vi "From Button Cluster To Button Table.vi"(8 "Error In":errorcluster, 11 "button info":T1) -> (0 "Error Out":errorcluster, 4 "Buttons array":bool[](array[boolean]), 5 "Which ones?":u8[](array[numeric]))   [LabVIEW 2014]
doc: "Converts buttons from joystick from cluster to table"
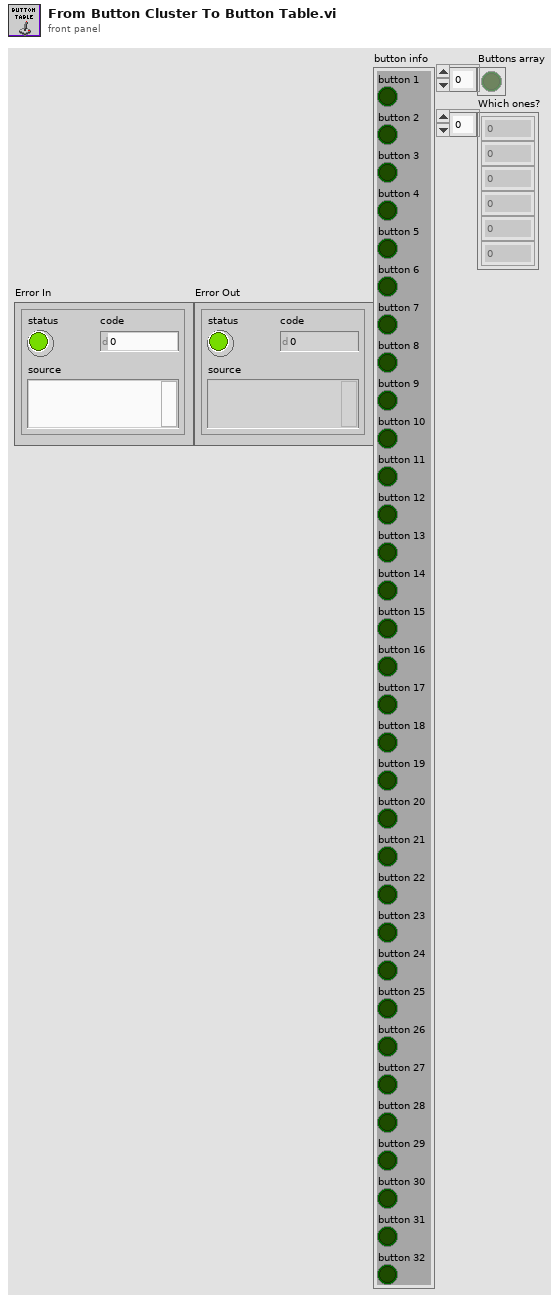
[diagram p1: front panel]
types:
  T1 = cluster{"button 1":bool, "button 2":bool, "button 3":bool, "button 4":bool, "button 5":bool, "button 6":bool, "button 7":bool, "button 8":bool, "button 9":bool, "button 10":bool, "button 11":bool, "button 12":bool, "button 13":bool, "button 14":bool, "button 15":bool, "button 16":bool, "button 17":bool, "button 18":bool, "button 19":bool, "button 20":bool, "button 21":bool, "button 22":bool, "button 23":bool, "button 24":bool, "button 25":bool, "button 26":bool, "button 27":bool, "button 28":bool, "button 29":bool, "button 30":bool, "button 31":bool, "button 32":bool}
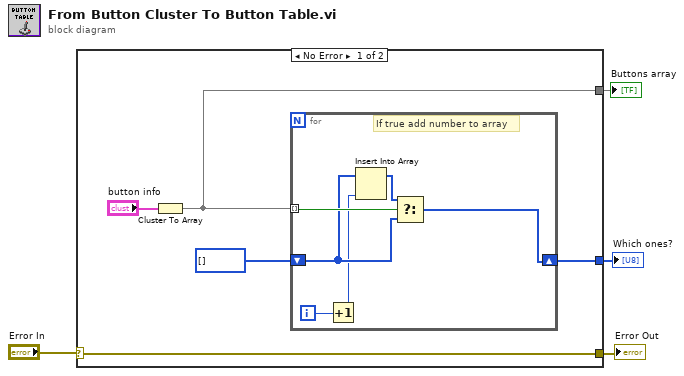
[diagram p0: block diagram]
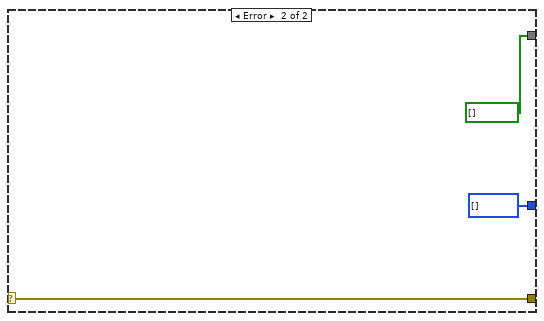
[diagram p2: hidden frame]
diagram:
  n1 = case shown="No Error" "Error In" {
    selector: "Error In" -> [w9 w18]
    tunnel: [w9 w18] -> w3
    tunnel: [w6 bool[] []] -> w2
    tunnel: [w5 u8[] []] -> w1
    frame No Error {
      n2 = Cluster To Array(cluster="button info") -> (array=w6:bool[])
      n3 = for {
        shift-right: [w14] -> w5
        shift-left: u8[] [] -> [w12]
        tunnel: w6 -> [w15] mode=indexing
        i -> [w13]
        # "If true add number to array"
        n4 = Increment(x=w13) -> (x+1=w11:i32)
        n5 = Insert Into Array(array=w12, new element=w11) -> (w10:u8[])  [unwired: 1 in]
        n6 = Select(t=w10, s=w15, f=w12) -> (s? t:f=w14:u8[])
      }
    }
    frame Error {
    }
  }
  "Error Out" <- w3
  "Buttons array" <- w2
  "Which ones?" <- w1
